vi "Zoom Window.vi"(7 "window size":i32, 8 "error in (no error)":errorcluster, 10 "Mouse Position":T1, 11 "CtlRef":refnum<vi>) -> (0 "error out":errorcluster)   [LabVIEW 2024]
uses:
  <vilib>/Utility/miscctls.llb/LVPoint32TypeDef.ctl
panel:
  out "Zoom Picture":picture
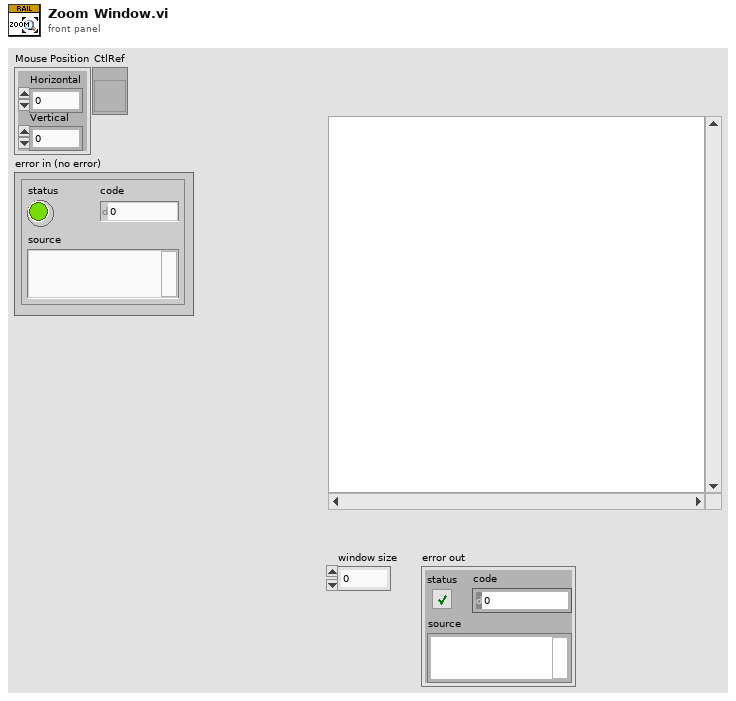
[diagram p1: front panel]
types:
  T1 = typedef "LVPoint32TypeDef.ctl" = cluster{"Horizontal":i32, "Vertical":i32}
  T2 = cluster{"Width":u16, "Style":enum32{"Solid", "Dash", "Dot", "DashDot", "DashDotDot"}}
  T3 = typedef "imagedata.ctl" = cluster{"image type":i32, "image depth":i32, "image":u8[], "mask":u8[], "colors":u32[], "Rectangle":cluster{"left":i16, "top":i16, "right":i16, "bottom":i16}}
  T4 = cluster{"[0]":dbl, "[1]":dbl, "[2]":dbl, "[3]":dbl}
  T5 = cluster{"left":i16, "top":i16, "right":i16, "bottom":i16}
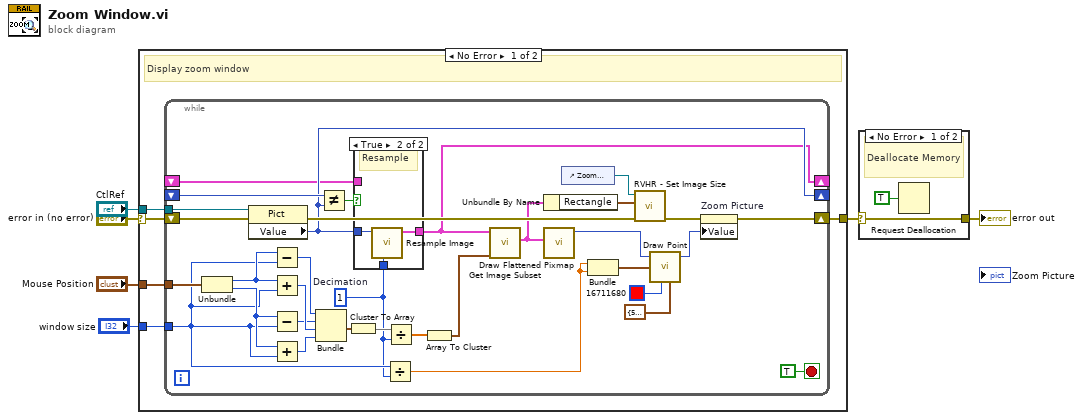
[diagram p0: block diagram]
diagram:
  n1 = case shown="No Error" "error in (no error)" {
    selector: "error in (no error)" -> [w11 w49]
    tunnel: "CtlRef" -> [w10 _]
    tunnel: "Mouse Position" -> [w9 _]
    tunnel: [w7 w49] -> w2
    tunnel: "window size" -> [w8 _]
    frame No Error {
      # "Display zoom window"
      n2 = while {
        tunnel: w10 -> [w43]
        tunnel: w9 -> [w42]
        tunnel: w8 -> [w18]
        shift-right: [w34] -> w7
        shift-left: w11 -> [w44]
        shift-right: [w16] -> _
        shift-left: _ -> [w32]
        shift-right: [w12] -> _
        shift-left: _ -> [w13]
        stop <- TRUE stop-if-true
        w15 = 1  # Decimation
        n3 = Unbundle(w42) -> ("Horizontal"=w41:i32, "Vertical"=w40:i32)
        n4 = property class="Pict"(reference=w43, error in=w44) -> (error out=w35:errorcluster, "Value"=w16:picture)  [unwired: 1 out]
        n5 = Subtract(x=w41, y=w18) -> (x-y=w39:i32)
        n6 = Add(x=w41, y=w18) -> (x+y=w38:i32)
        n7 = Subtract(x=w40, y=w18) -> (x-y=w36:i32)
        n8 = Add(x=w40, y=w18) -> (x+y=w37:i32)
        n9 = Bundle(w39, w36, w38, w37) -> (w25:cluster{i32, i32, i32, i32})  [unwired: 1 in]
        n10 = Not Equal?(x=w32, y=w16) -> (x != y?=w14:bool)
        n11 = Cluster To Array(cluster=w25) -> (array=w26:i32[])
        n12 = case shown="True" w14 {
          tunnel: w16 -> [_ w48]
          tunnel: [w45 w47] -> w12
          tunnel: w15 -> [_ w46]
          tunnel: w13 -> [w45 _]
          frame False {
          }
          frame True {
            # "Resample"
            n13 = call "Resample Image.vi"("Decimation"=w46, "Picture"=w48) -> ("image data"=w47:T3)  [unwired: 9 in]
          }
        }
        n14 = Divide(x=w18, y=w15) -> (x/y=w17:dbl)
        n15 = Divide(x=w26, y=w15) -> (x/y=w27:dbl[])
        n16 = Array To Cluster(array=w27) -> (cluster=w24:T4)
        n17 = call <vilib>:"Get Image Subset.vi"("subset rect"=w24, "image data"=w12) -> ("image subset"=w31:T3)  [unwired: 4 in, 1 out]
        n18 = Unbundle By Name(w31) -> ("Rectangle"=w30:T5)
        n19 = call <vilib>:"Draw Flattened Pixmap.vi"("image data"=w31) -> ("new picture"=w20:picture)  [unwired: 8 in]
        n20 = control-ref of="Zoom Picture"() -> (w29:refnum<vi>)
        n21 = Bundle(w17, w17) -> (w23:cluster{dbl, dbl})  [unwired: 1 in]
        n22 = call "RVHR - Set Image Size.vi"("error in (no error)"=w35, "Rectangle"=w30, "Image_L"=w29) -> ("error out"=w28:errorcluster)  [unwired: 8 in]
        n23 = call <vilib>:"Draw Point.vi"("picture"=w20, "point(x,y)"=w23, "color(black)"=u32 16711680, "pen"=T2 {"Width"=5, "Style"=enum."Solid"}) -> ("new picture"=w19:picture)  [unwired: 5 in]
        n24 = property on="Zoom Picture" class="Pict"(error in=w28, "Value"=w19) -> (error out=w34:errorcluster)  [unwired: 1 in, 1 out]
      }
    }
    frame Error {
    }
  }
  n25 = case shown="No Error" w2 {
    selector: w2 -> [w50 w52]
    tunnel: [w50 w52] -> w1
    frame No Error {
      # "Deallocate Memory"
      n26 = Request Deallocation(TRUE ("flag")) -> ()
    }
    frame Error {
    }
  }
  "error out" <- w1
